vi "string length.vi"() -> ()   [LabVIEW 2020]
panel:
  out "Slide":i32(slide) scale=0.0..50.0
  out "length":i32
  in  "String":string="sanket"
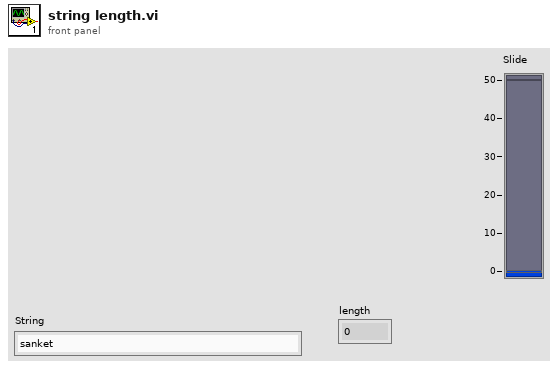
[diagram p1: front panel]
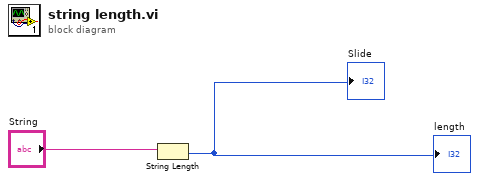
[diagram p0: block diagram]
diagram:
  n1 = String Length(string="String") -> (length=→"length" →"Slide":i32)
